vi "Example Multiplex Server.vi"() -> ()   [LabVIEW 2020]
uses:
  <vilib>/gpm_packages/@cs/event-logger/Source/Composed Log/LoggerReference/LoggerReference.lvclass/LoggerReference.ctl
  <vilib>/gpm_packages/@cs/Network-interface/Source/Network Messenger/Header Data Packet Return/Header Data Packet Return.lvclass/Header Data Packet Return.ctl
  <vilib>/gpm_packages/@cs/Network-interface/Source/Network Messenger/Multiplexed Messenger/Multiplexed Messenger.lvclass/Multiplexed Messenger.ctl
  <vilib>/gpm_packages/@cs/Network-interface/Source/Create Ref Message/Create Ref Message.lvclass/Create Ref Message.ctl
  <vilib>/ActorFramework/Message Enqueuer/Message Enqueuer.lvclass/Message Enqueuer.ctl
  <vilib>/gpm_packages/@cs/Network-interface/Examples/Client Actor/Client Actor/Client Actor.lvclass
  C:/Program Files/National Instruments/LabVIEW 2020/vi.lib/ActorFramework/Actor/Actor.lvclass
  <vilib>/gpm_packages/@cs/Network-interface/Source/Network Messenger/Synchronous Write Callback/Synchronous Write Callback.lvclass/Synchronous Write Callback.ctl
  <vilib>/gpm_packages/@cs/Network-interface/Source/MessagingInterfaces/WriteRequest/WriteRequest.lvclass/WriteRequest.ctl
  <vilib>/gpm_packages/@cs/Network-interface/Source/MultiplexedConnectionHandler/MultiplexedConnectionHandler Messages/Execute Single Point Write Request Msg/Execute Single Point Write Request Msg.lvclass/Execute Single Point Write Request Msg.ctl
  <vilib>/gpm_packages/@cs/Network-interface/Source/PersistantConnectionHandler/PersistantConnectionHandler Messages/Execute Write Request Msg/Execute Write Request Msg.lvclass/Execute Write Request Msg.ctl
  166efa5d-3c92-4a7f-98b7-f33b376e2f94.vi
  <vilib>/gpm_packages/@cs/event-logger/Source/Composed Log/LoggerReference/Return Aggregate Queues.vi
  <vilib>/gpm_packages/@cs/event-logger/Source/Composed Log/LoggerReference/Add Aggregate Log.vi
  166efa5d-3c92-4a7f-98b7-f33b376e2f94.vi/35e97c32-9302-4122-b064-4effb2cc8bb9.vi
  <vilib>/gpm_packages/@cs/Network-interface/Source/Create Ref Message/Send Create Reference Message and Wait On Return.vi
  <vilib>/gpm_packages/@cs/Network-interface/Source/Network Messenger/Header Data Packet Return/Construct Header Data Packet Return.vi
  <vilib>/gpm_packages/@cs/Network-interface/Source/MessagingInterfaces/WriteRequest/Pack Write Request.vi
  <vilib>/gpm_packages/@cs/Network-interface/Source/Network Messenger/Synchronous Write Callback/Construct.vi
  <vilib>/gpm_packages/@cs/Network-interface/Source/Network Messenger/Synchronous Write Callback/Wait On Execution.vi
  <vilib>/gpm_packages/@cs/Network-interface/Source/MultiplexedConnectionHandler/MultiplexedConnectionHandler Messages/Execute Single Point Write Request Msg/Send Execute Single Point Write Request.vi
  <vilib>/gpm_packages/@cs/Network-interface/Source/PersistantConnectionHandler/PersistantConnectionHandler Messages/Execute Write Request Msg/Send Execute Write Request.vi
  <vilib>/ActorFramework/Message Enqueuer/Enqueue.vi
  <vilib>/gpm_packages/@cs/event-logger/Source/Composed Log/LoggerReference/Send Add Sink.vi
  <vilib>/gpm_packages/@cs/Network-interface/Examples/EventConnectionCallback/EventConnectionCallback.lvclass
  C:/Program Files/National Instruments/LabVIEW 2020/vi.lib/gpm_packages/@cs/Network-interface/Source/MessagingInterfaces/IConnectionStateChangeCallback/IConnectionStateChangeCallback.lvclass
  <vilib>/gpm_packages/@cs/event-logger/Source/String Control Sink/String Control Sink.lvclass
  C:/Program Files/National Instruments/LabVIEW 2020/vi.lib/gpm_packages/@cs/event-logger/Source/Composed Log/Log Sink/Log Sink.lvclass
  <vilib>/gpm_packages/@cs/Network-interface/Examples/EventMessageRxCallback/EventMessageRxCallback.lvclass
  C:/Program Files/National Instruments/LabVIEW 2020/vi.lib/gpm_packages/@cs/Network-interface/Source/Network Messenger/IPacket Return/IPacket Return.lvclass
  <vilib>/gpm_packages/@cs/Network-interface/Source/Network Messenger/Write Strategy/Write Strategy.lvclass
  C:/Program Files/National Instruments/LabVIEW 2020/vi.lib/gpm_packages/@cs/Network-interface/Source/MessagingInterfaces/IWriteStrategy/IWriteStrategy.lvclass
  <vilib>/gpm_packages/@cs/Network-interface/Source/Network Messenger/ReadStrategy/ReadStrategy.lvclass
  C:/Program Files/National Instruments/LabVIEW 2020/vi.lib/gpm_packages/@cs/Network-interface/Source/MessagingInterfaces/IReadStrategy/IReadStrategy.lvclass
  <vilib>/gpm_packages/@cs/Network-interface/Source/MultiplexedConnectionHandler/MultiplexedConnectionHandler/MultiplexedConnectionHandler.lvclass
  C:/Program Files/National Instruments/LabVIEW 2020/vi.lib/gpm_packages/@cs/Network-interface/Source/PersistantConnectionHandler/PersistantConnectionHandler/PersistantConnectionHandler.lvclass
  <vilib>/gpm_packages/@cs/Network-interface/Source/Network Messenger/Header Data Packet Return/Header Data Packet Return.lvclass
  C:/Program Files/National Instruments/LabVIEW 2020/vi.lib/gpm_packages/@cs/Network-interface/Source/MessagingInterfaces/IMessageReturnPolicy/IMessageReturnPolicy.lvclass
  <vilib>/gpm_packages/@cs/Network-interface/Source/TCP Interface/TCP Server/TCP Server.lvclass
  C:/Program Files/National Instruments/LabVIEW 2020/vi.lib/gpm_packages/@cs/Network-interface/Source/IConnectionFactory/IConnectionFactory.lvclass
  <vilib>/gpm_packages/@cs/Network-interface/Source/Create Ref Message/Create Ref Message.lvclass
  C:/Program Files/National Instruments/LabVIEW 2020/vi.lib/ActorFramework/Message/Message.lvclass
  <vilib>/gpm_packages/@cs/Network-interface/Source/Network Messenger/Synchronous Write Callback/Synchronous Write Callback.lvclass
  C:/Program Files/National Instruments/LabVIEW 2020/vi.lib/gpm_packages/@cs/Network-interface/Source/MessagingInterfaces/IWriteExecutionCallback/IWriteExecutionCallback.lvclass
  <vilib>/gpm_packages/@cs/Network-interface/Source/Network Messenger/ClusterMessagePacket/ClusterMessagePacket.lvclass
  C:/Program Files/National Instruments/LabVIEW 2020/vi.lib/gpm_packages/@cs/Network-interface/Source/MessagingInterfaces/IPacket/IPacket.lvclass
  <vilib>/gpm_packages/@cs/Network-interface/Source/MultiplexedConnectionHandler/MultiplexedConnectionHandler Messages/Execute Single Point Write Request Msg/Execute Single Point Write Request Msg.lvclass
  <vilib>/gpm_packages/@cs/Network-interface/Source/PersistantConnectionHandler/PersistantConnectionHandler Messages/Execute Write Request Msg/Execute Write Request Msg.lvclass
  <vilib>/ActorFramework/Stop Msg/Stop Msg.lvclass
  <vilib>/gpm_packages/@cs/event-logger/Source/Composed Log/Application Logger/Launch Worker Loop.vi
  <vilib>/gpm_packages/@cs/event-logger/Source/Composed Log/LoggerReference/Initialize Logger Instance.vi
  <vilib>/gpm_packages/@cs/Network-interface/Source/MultiplexedConnectionHandler/MultiplexedConnectionHandler/Set Number Of Connections To Make.vi
  <vilib>/gpm_packages/@cs/Network-interface/Source/TCP Interface/TCP Server/Construct TCP Server.vi
  <vilib>/gpm_packages/@cs/Network-interface/Source/PersistantConnectionHandler/PersistantConnectionHandler/Pack Connection Handler.vi
  <vilib>/ActorFramework/Message Priority Queue/Priority Enqueue.vi
  <vilib>/gpm_packages/@cs/Network-interface/Source/Network Messenger/ClusterMessagePacket/Pack.vi
  <vilib>/gpm_packages/@cs/event-logger/Source/Composed Log/LoggerReference/LoggerReference.lvclass
  <vilib>/gpm_packages/@cs/event-logger/Source/Composed Log/IErrorFormat/IErrorFormat.lvclass
  <vilib>/gpm_packages/@cs/event-logger/Source/Composed Log/Log Sink/Log Sink.lvclass
  <vilib>/gpm_packages/@cs/Network-interface/Source/Network Messenger/Multiplexed Messenger/Multiplexed Messenger.lvclass
  <vilib>/gpm_packages/@cs/Network-interface/Source/MessagingInterfaces/WriteRequest/WriteRequest.lvclass
  <vilib>/ActorFramework/Message Enqueuer/Message Enqueuer.lvclass
  <vilib>/ActorFramework/Actor/Actor.lvclass
panel:
  out "Message Log":string
  in  "Send to Unique":bool
  in  "Send to All":bool
  in  "Message To Send":string
  in  "Spawn New Connection":bool
  in  "Active Connections":i32(listbox)
  in  "Event Log":string
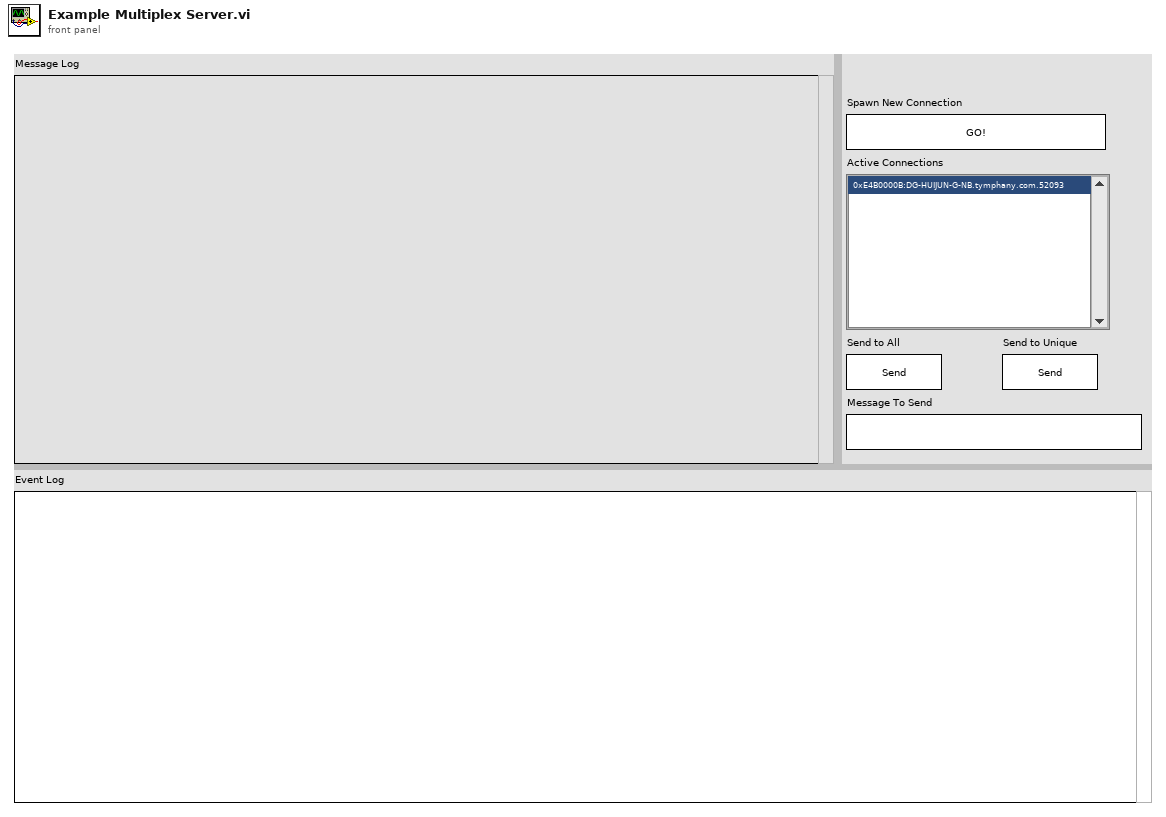
[diagram p1: front panel]
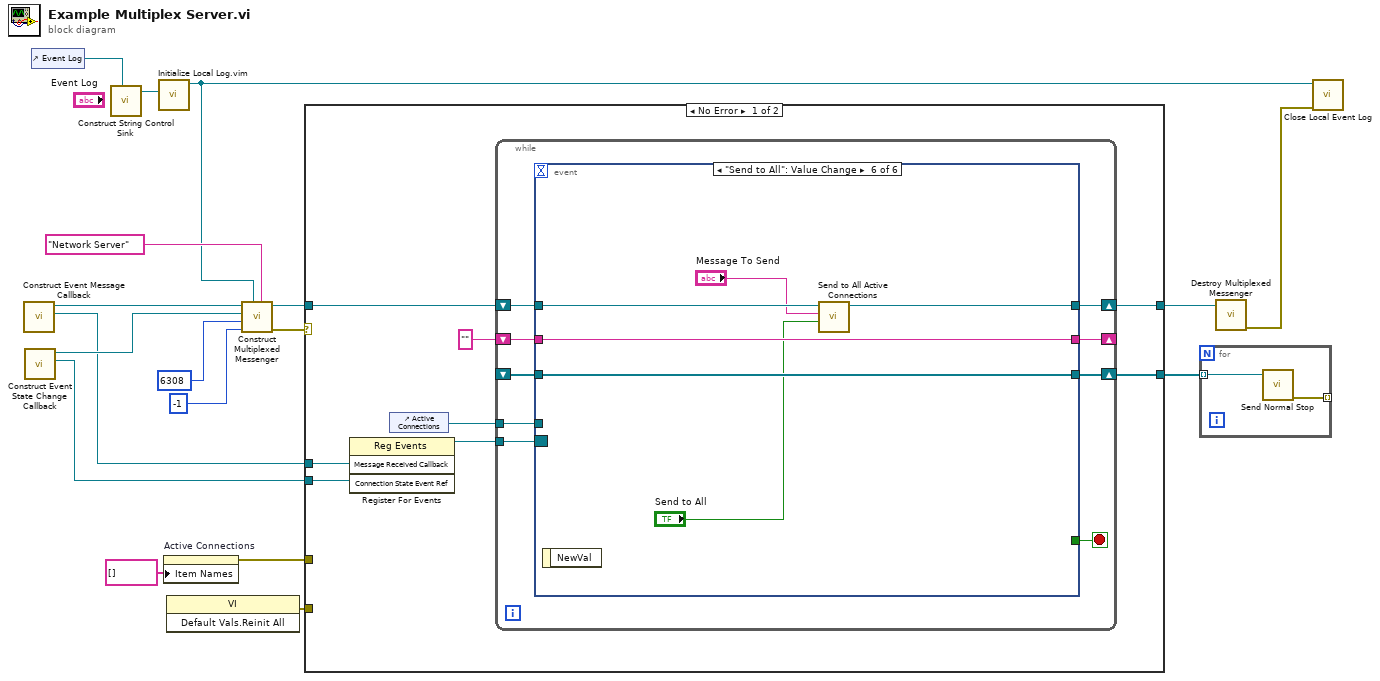
[diagram p0: block diagram]
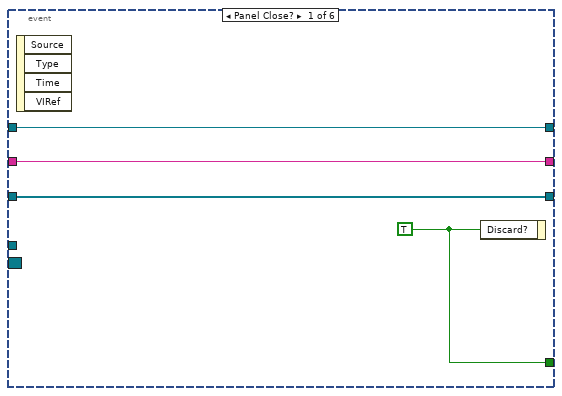
[diagram p2: hidden frame]
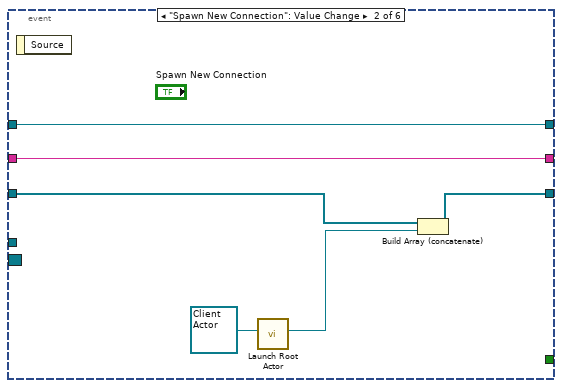
[diagram p3: hidden frame]
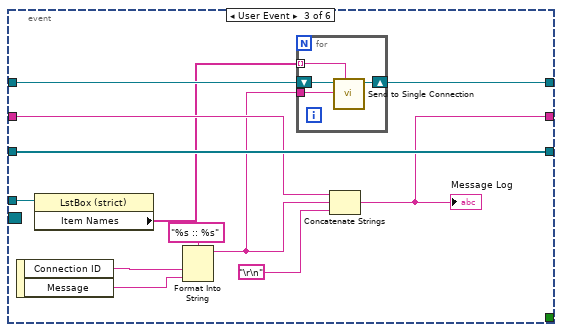
[diagram p4: hidden frame]
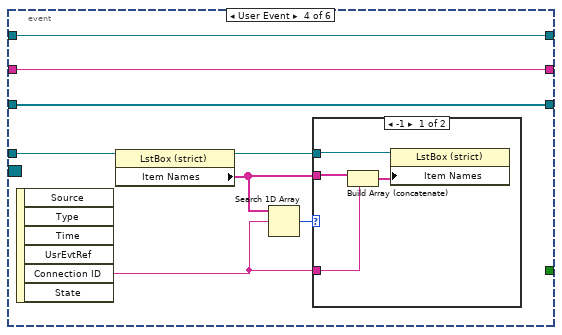
[diagram p5: hidden frame]
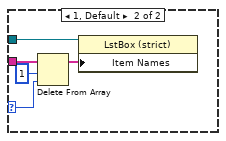
[diagram p6: hidden frame]
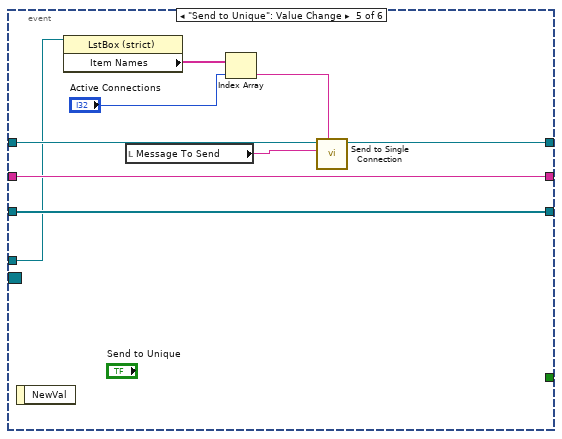
[diagram p7: hidden frame]
diagram:
  n1 = call <vilib>:"Construct Event Message Callback.vi"() -> ("Message Received Callback"=w11:refnum<user-event>, "EventMessageRxCallback out"=w12:refnum<class "EventMessageRxCallback.lvclass">)  [unwired: 9 in, 1 out]
  n2 = call <vilib>:"Construct Event State Change Callback.vi"() -> ("Connection State Event Ref"=w1:refnum<user-event>, "EventConnectionCallback out"=w13:refnum<class "EventConnectionCallback.lvclass">)  [unwired: 9 in, 1 out]
  n3 = control-ref of="Event Log"() -> (w15:refnum<vi>)
  n4 = call <vilib>:"Construct String Control Sink.vi"("Str Refnum"=w15) -> ("String Control Sink out"=w16:refnum<class "String Control Sink.lvclass">)  [unwired: 10 in]
  n5 = call "Initialize Local Log.vim"("Startup Sink(s)"=w16) -> ("Log Instance Reference"=w7:refnum<class "LoggerReference.lvclass">)  [unwired: 8 in, 2 out]
  n6 = property on="Active Connections" class="LstBox (strict)"("Item Names"=string[] []) -> (error out=w4:errorcluster)  [unwired: 2 in, 1 out]
  n7 = invoke class="VI" method="Default Vals.Reinit All"() -> (error out=w2:errorcluster)  [unwired: 3 in, 2 out]
  n8 = call <vilib>:"Construct Multiplexed Messenger.vi"("Log Alias"="Network Server", "Log Instance"=w7, "Connections To Make"=-1, "Port"=u16 6308, "Connection State Change Callback"=w13, "Packet Return"=w12) -> ("error out"=w10:errorcluster, "Multiplexed Messenger Out"=w9:refnum<data-value>)  [unwired: 4 in]
  n9 = case shown="No Error" w10 {
    tunnel: w11 -> [w26 _]
    tunnel: w1 -> [w25 _]
    tunnel: w9 -> [w23 w94]
    tunnel: [w22 w94] -> w8
    tunnel: [w21 _] -> w5
    tunnel: w4 -> [_ _]
    tunnel: w2 -> [_ _]
    frame No Error {
      n10 = register-events(w26, w25) -> (reference out=w24:refnum<event-registration>)  [unwired: 2 in, 1 out]
      n11 = control-ref of="Active Connections"() -> (w19:refnum<vi>)
      n12 = while {
        tunnel: w24 -> [w35]
        shift-right: [w33] -> w22
        shift-left: w23 -> [w34]
        shift-right: [w31] -> w21
        shift-left: _ -> [w30]
        shift-right: [w28] -> _
        shift-left: "" -> [w29]
        tunnel: w19 -> [w27]
        stop <- w32 stop-if-true
        n13 = event shown="[5] \"Send to All\": Value Change" {
          selector: w35 -> [_ _ _ _ _ _]
          dyn-events: _ -> [_ _ _ _ _ _]
          timeout: _ -> [_ _ _ _ _ _]
          tunnel: w34 -> [w38 w45 w50 w69 w85 w91]
          tunnel: [w38 w45 w49 w69 w84 w90] -> w33
          tunnel: [w39 _ _ _ _ _] -> w32
          tunnel: [w37 w42 w57 w68 w87 w93] -> w31
          tunnel: w30 -> [w37 w41 w57 w68 w87 w93]
          tunnel: w29 -> [w36 w40 w53 w67 w86 w92]
          tunnel: [w36 w40 w52 w67 w86 w92] -> w28
          tunnel: w27 -> [_ _ w51 w62 w83 _]
          event Panel Close? {
            w39 = TRUE ("Discard?")
            n14 = event-data() -> ()  [unwired: 1 in, 4 out]
            n15 = event-data("Discard?"=w39) -> ()  [unwired: 1 in, 1 out]
          }
          event "Spawn New Connection": Value Change {
            n16 = event-data() -> ()  [unwired: 1 in, 1 out]
            n17 = call <vilib>:"Launch Root Actor.vi"("Actor"=refnum<class "Client Actor.lvclass"> refnum ("Client Actor.lvlib:Client Actor.lvclass")) -> ("Actor's Enqueuer"=w43:refnum<class "Message Enqueuer.lvclass">)  [unwired: 9 in, 1 out]
            n18 = Build Array (concatenate)(w41, w43) -> (w42:refnum<class "Message Enqueuer.lvclass">[])
          }
          event User Event {
            n19 = event-data() -> ("Connection ID"=w56:string, "Message"=w55:string)  [unwired: 1 in]
            n20 = property on="Property Node" class="LstBox (strict)"(reference=w51) -> ("Item Names"=w48:string[])  [unwired: 1 in, 2 out]
            n21 = Format Into String(format string="%s :: %s", w56, w55) -> (resulting string=w47:string)  [unwired: 2 in, 1 out]
            n22 = for {
              shift-right: [w60] -> w49
              shift-left: w50 -> [w61]
              tunnel: w48 -> [w59] mode=indexing
              tunnel: w47 -> [w58]
              n23 = call <vilib>:"Send to Single Connection.vi"("Connection ID"=w59, "Message"=w58, "Multiplexed Messenger In"=w61) -> ("Multiplexed Messenger Out"=w60:refnum<data-value>)  [unwired: 7 in, 1 out]
            }
            n24 = Concatenate Strings(w53, w47, "\r\n") -> (w52:string)
            "Message Log" <- w52
          }
          event User Event {
            n25 = event-data() -> ("Connection ID"=w63:string)  [unwired: 1 in, 5 out]
            n26 = property class="LstBox (strict)"(reference=w62) -> (reference out=w64:refnum<vi>, "Item Names"=w65:string[])  [unwired: 1 in, 1 out]
            n27 = Search 1D Array(1D array=w65, element=w63) -> (index of element=w66:i32)  [unwired: 1 in]
            n28 = case shown="-1" w66 {
              selector: w66 -> [_ w76]
              tunnel: w65 -> [w72 w77]
              tunnel: w64 -> [w73 w78]
              tunnel: w63 -> [w70 _]
              frame -1 {
                n29 = Build Array (concatenate)(w72, w70) -> (w71:string[])
                n30 = property class="LstBox (strict)"(reference=w73, "Item Names"=w71) -> ()  [unwired: 1 in, 2 out]
              }
              frame 1, Default {
                n31 = Delete From Array(array=w77, length=1, index=w76) -> (array with subset deleted=w75:string[])  [unwired: 1 out]
                n32 = property class="LstBox (strict)"(reference=w78, "Item Names"=w75) -> ()  [unwired: 1 in, 2 out]
              }
            }
          }
          event "Send to Unique": Value Change {
            n33 = event-data() -> ()  [unwired: 1 in, 1 out]
            n34 = property on="Property Node" class="LstBox (strict)"(reference=w83) -> ("Item Names"=w82:string[])  [unwired: 1 in, 2 out]
            n35 = local read "Message To Send"() -> (w79:string)
            n36 = Index Array(array=w82, index="Active Connections") -> (element=w80:string)
            n37 = call <vilib>:"Send to Single Connection.vi"("Connection ID"=w80, "Message"=w79, "Multiplexed Messenger In"=w85) -> ("Multiplexed Messenger Out"=w84:refnum<data-value>)  [unwired: 7 in, 1 out]
          }
          event "Send to All": Value Change {
            n38 = event-data() -> ()  [unwired: 1 in, 1 out]
            n39 = call <vilib>:"Send to All Active Connections.vi"("Data"="Send to All", "Message"="Message To Send", "Multiplexed Messenger In"=w91) -> ("Multiplexed Messenger Out"=w90:refnum<data-value>)  [unwired: 7 in, 1 out]
          }
        }
      }
    }
    frame Error {
    }
  }
  n40 = for {
    tunnel: w5 -> [w96] mode=indexing
    tunnel: [w95] -> _ mode=indexing
    n41 = call <vilib>:"Send Normal Stop.vi"("Message Enqueuer"=w96) -> ("error out"=w95:errorcluster)  [unwired: 10 in]
  }
  n42 = call <vilib>:"Destroy Multiplexed Messenger.vi"("Multiplexed Messenger In"=w8) -> ("error out"=w6:errorcluster)  [unwired: 10 in]
  n43 = call <vilib>:"Close Local Event Log.vi"("error in (no error)"=w6, "Log Instance"=w7) -> ()  [unwired: 9 in, 1 out]
